vi "Resource Name Empty Check.vi"(8 "error in (no error)":errorcluster, 11 "RESOURCE NAME Ref":refnum<vi>) -> (0 "error out":errorcluster, 3 "RESOURCE NAME Ref out":refnum<vi>)   [LabVIEW 2025, in "I2C Bus Monitor UI.lvlib"]
uses:
  I2C Bus Monitor UI.lvlib
  Error Global.vi
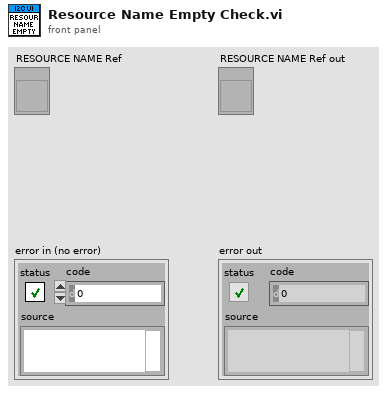
[diagram p1: front panel]
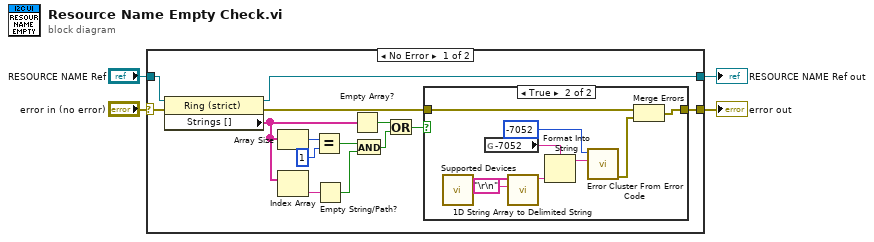
[diagram p0: block diagram]
diagram:
  n1 = case shown="No Error" "error in (no error)" {
    selector: "error in (no error)" -> [w16 w29]
    tunnel: "RESOURCE NAME Ref" -> [w18 w30]
    tunnel: [w17 w30] -> w3
    tunnel: [w14 w29] -> w1
    frame No Error {
      n2 = property on="Property Node" class="Ring (strict)"(reference=w18, error in=w16) -> (reference out=w17:refnum<vi>, error out=w15:errorcluster, "Strings []"=w8:string[])
      n3 = Array Size(array=w8) -> (size(s)=w10:i32)
      n4 = Index Array(array=w8) -> (element=w7:string)  [unwired: 1 in]
      n5 = Equal?(x=w10, y=1 ("x")) -> (x = y?=w5:bool)
      n6 = Empty String/Path?(string/path=w7) -> (empty?=w6:bool)
      n7 = Empty Array?(array=w8) -> (empty?=w13:bool)
      n8 = And(x=w5, y=w6) -> (x .and. y?=w11:bool)
      n9 = Or(x=w13, y=w11) -> (x .or. y?=w12:bool)
      n10 = case shown="True" w12 {
        tunnel: w15 -> [w19 w22]
        tunnel: [w19 w21] -> w14
        frame False {
        }
        frame True {
          n11 = call "Supported Devices.vi"() -> ("Supported Devices"=w23:string[])  [unwired: 11 in]
          n12 = global read "Error Global.vi" "-7052"() -> (w26:string)
          n13 = call <vilib>:"1D String Array to Delimited String.vi"("delimiter"="\r\n", "string array"=w23) -> ("delimited string"=w27:string)  [unwired: 9 in]
          n14 = Format Into String(format string=w26, w27) -> (resulting string=w28:string)  [unwired: 2 in, 1 out]
          n15 = call <vilib>:"Error Cluster From Error Code.vi"("error message (\"\")"=w28, "error code (0)"=-7052) -> ("error out"=w20:errorcluster)  [unwired: 7 in]
          n16 = Merge Errors(w22, w20) -> (w21:errorcluster)
        }
      }
    }
    frame Error {
    }
  }
  "error out" <- w1
  "RESOURCE NAME Ref out" <- w3
